vi "get_ROIs_in_um.vi"(4 "error in (no error)":errorcluster, 6 "Container State":T10, 7 "Display State In":T1={"current frame index"=0, "number of images"=0, "ROI (frames)"={"ROI"=[]}, "control refs"={"frame"=refnum, "image"=refnum, "saveROIsButton"=refnum, "loadImageSwitch"=refnum, "loadROIsSwitch"=refnum, "saveROIsSwitch"=refnum, "loadImagePath"=refnum, "loadROIPath"=refnum, "redraw"=refnum}, "calibration"={"x"=0.0, "y"=0.0, "x unit"=enum."um", "y unit"=enum."um"}, "xpaths"={"x offset"="", "y offset"="", "z offset"=""}, "offset"=refnum, "XML description"="", "number of ROIs"=0.0, "ROI Tool Buttons Visible"={"Zoom Tool"=TRUE, "Selection Tool"=TRUE, "Pan Tool"=TRUE, "Point Tool"=TRUE, "Line Tool"=TRUE, "Rectangle Tool"=TRUE, "Rotated Rectangle Tool"=TRUE, "Polyline Tool"=TRUE, "Polygon Tool"=TRUE, "Freehand Tool"=TRUE, "Closed Freehand Tool"=TRUE, "Ellipse Tool"=TRUE, "Annulus Tool"=TRUE}, "ROI color"=6618880, "number color"=6618880, "enable ROI numbering?"=FALSE, "selected path to save ROIs"=path "", "starting path"=path "", "array of overlays"=[], "pointCollection"=refnum, "ROImode"=enum."IMAQROIs", "selected point ID"=0.0, "point radius"=5, "point colours"=[], "PlotAreaSize"={"Width"=0, "Height"=0}, "last action"=enum."not specified"} {"array of overlays"."overlay size" min=1}) -> (0 "error out":errorcluster, 2 "Value":T11, 3 "Display State Out":T1={"current frame index"=0, "number of images"=0, "ROI (frames)"={"ROI"=[]}, "control refs"={"frame"=refnum, "image"=refnum, "saveROIsButton"=refnum, "loadImageSwitch"=refnum, "loadROIsSwitch"=refnum, "saveROIsSwitch"=refnum, "loadImagePath"=refnum, "loadROIPath"=refnum, "redraw"=refnum}, "calibration"={"x"=0.0, "y"=0.0, "x unit"=enum."um", "y unit"=enum."um"}, "xpaths"={"x offset"="", "y offset"="", "z offset"=""}, "offset"=refnum, "XML description"="", "number of ROIs"=0.0, "ROI Tool Buttons Visible"={"Zoom Tool"=TRUE, "Selection Tool"=TRUE, "Pan Tool"=TRUE, "Point Tool"=TRUE, "Line Tool"=TRUE, "Rectangle Tool"=TRUE, "Rotated Rectangle Tool"=TRUE, "Polyline Tool"=TRUE, "Polygon Tool"=TRUE, "Freehand Tool"=TRUE, "Closed Freehand Tool"=TRUE, "Ellipse Tool"=TRUE, "Annulus Tool"=TRUE}, "ROI color"=6618880, "number color"=6618880, "enable ROI numbering?"=FALSE, "selected path to save ROIs"=path "", "starting path"=path "", "array of overlays"=[], "pointCollection"=refnum, "ROImode"=enum."IMAQROIs", "selected point ID"=0.0, "point radius"=5, "point colours"=[], "PlotAreaSize"={"Width"=0, "Height"=0}, "last action"=enum."not specified"} {"array of overlays"."overlay size" min=1})   [LabVIEW 2010, in "XImage.xctl"]
uses:
  XImage.xctl
  <vilib>/_xctls/Container State.ctl
  ROImicrons_frames_cluster.ctl
  ROImicrons_cluster.ctl
  state.ctl
  classes/SpaceVector/SpaceVector/SpaceVector.lvclass
  classes/PointCollection/PointCollection/PointCollection.lvclass
  ROI_frames_cluster.ctl
  control_refs_cluster.ctl
  calibration_cluster.ctl
  enumerations/unit.ctl
  xpath_cluster.ctl
  overlays_cluster.ctl
  ROI_mode_enum.ctl
  last_action_enum.ctl
  <vilib>/_xctls/XControlSupport.lvlib
  classes/Image/Image/Image.lvclass
panel:
  # "Replace the Value Indicator below with an Indicator of desired type.\nDo not remove this Indicator or the others from the connector pane. \nDo not change the connector pane pattern.\nThe Value Indicator should always be the second terminal from top on the output side in the connector pane."
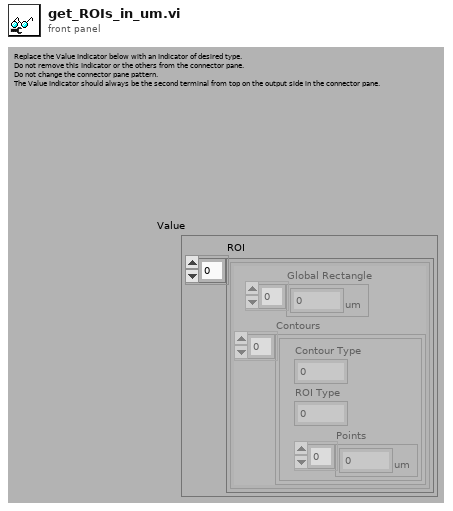
[diagram p1: front panel]
types:
  T1 = typedef "XImage.xctl/state.ctl" = cluster{"current frame index":i32, "number of images":i32, "ROI (frames)":T2, "control refs":T3, "calibration":T4, "xpaths":T6, "offset":refnum<class "SpaceVector.lvclass">, "XML description":string, "number of ROIs":dbl, "ROI Tool Buttons Visible":cluster{"Zoom Tool":bool, "Selection Tool":bool, "Pan Tool":bool, "Point Tool":bool, "Line Tool":bool, "Rectangle Tool":bool, "Rotated Rectangle Tool":bool, "Polyline Tool":bool, "Polygon Tool":bool, "Freehand Tool":bool, "Closed Freehand Tool":bool, "Ellipse Tool":bool, "Annulus Tool":bool}, "ROI color":u32, "number color":u32, "enable ROI numbering?":bool, "selected path to save ROIs":path, "starting path":path, "array of overlays":T7[], "pointCollection":refnum<class "PointCollection.lvclass">, "ROImode":T8, "selected point ID":dbl, "point radius":i32, "point colours":u32[], "PlotAreaSize":cluster{"Width":u32, "Height":u32}, "last action":T9}
  T2 = typedef "XImage.xctl/ROI_frames_cluster.ctl" = cluster{"ROI":cluster{"Global Rectangle":i32[], "Contours":cluster{"Contour Type":u32, "ROI Type":u32, "Points":i32[]}[]}[]}
  T3 = typedef "XImage.xctl/control_refs_cluster.ctl" = cluster{"frame":refnum<vi>, "image":refnum<vi>, "saveROIsButton":refnum<vi>, "loadImageSwitch":refnum<vi>, "loadROIsSwitch":refnum<vi>, "saveROIsSwitch":refnum<vi>, "loadImagePath":refnum<vi>, "loadROIPath":refnum<vi>, "redraw":refnum<vi>}
  T4 = typedef "XImage.xctl/calibration_cluster.ctl" = cluster{"x":dbl, "y":dbl, "x unit":T5, "y unit":T5}
  T5 = typedef "Image.lvclass/unit.ctl" = enum16{"um", "s"}
  T6 = typedef "XImage.xctl/xpath_cluster.ctl" = cluster{"x offset":string, "y offset":string, "z offset":string}
  T7 = typedef "XImage.xctl/overlays_cluster.ctl" = cluster{"overlay array":cluster{i32[][]}[], "overlay name":string, "color (red)":u32, "overlay size":i32, "overlay type":enum16{"crosshair", "circle"}}
  T8 = typedef "XImage.xctl/ROI_mode_enum.ctl" = enum16{"none", "IMAQROIs", "PointCollection"}
  T9 = typedef "XImage.xctl/last_action_enum.ctl" = enum16{"not specified", "image loaded", "frame changed", "ROIs changed"}
  T10 = typedef "XControlSupport.lvlib/Container State.ctl" = cluster{"Indicator?":bool, "Run Mode?":bool, " Refnum":refnum<vi>}
  T11 = typedef "XImage.xctl/ROImicrons_frames_cluster.ctl" = cluster{"ROI":T12[]}
  T12 = typedef "ROImicrons_cluster.ctl" = cluster{"Global Rectangle":dbl[unit][], "Contours":cluster{"Contour Type":u32, "ROI Type":u32, "Points":dbl[unit][]}[]}
  T13 = cluster{"Global Rectangle":dbl[unit][], "Contours":cluster{"Contour Type":u32, "ROI Type":u32, "Points":dbl[unit][]}[]}
  T14 = cluster{"Contour Type":u32, "ROI Type":u32, "Points":dbl[unit][]}
  T15 = cluster{"Global Rectangle":i32[], "Contours":cluster{"Contour Type":u32, "ROI Type":u32, "Points":i32[]}[]}[]
  T16 = cluster{"Global Rectangle":dbl[unit][], "Contours":cluster{"Contour Type":u32, "ROI Type":u32, "Points":dbl[unit][]}[]}[]
  T17 = cluster{"Contour Type":u32, "ROI Type":u32, "Points":i32[]}[]
  T18 = cluster{"[0]":dbl, "[1]":dbl, "[2]":dbl, "[3]":dbl}
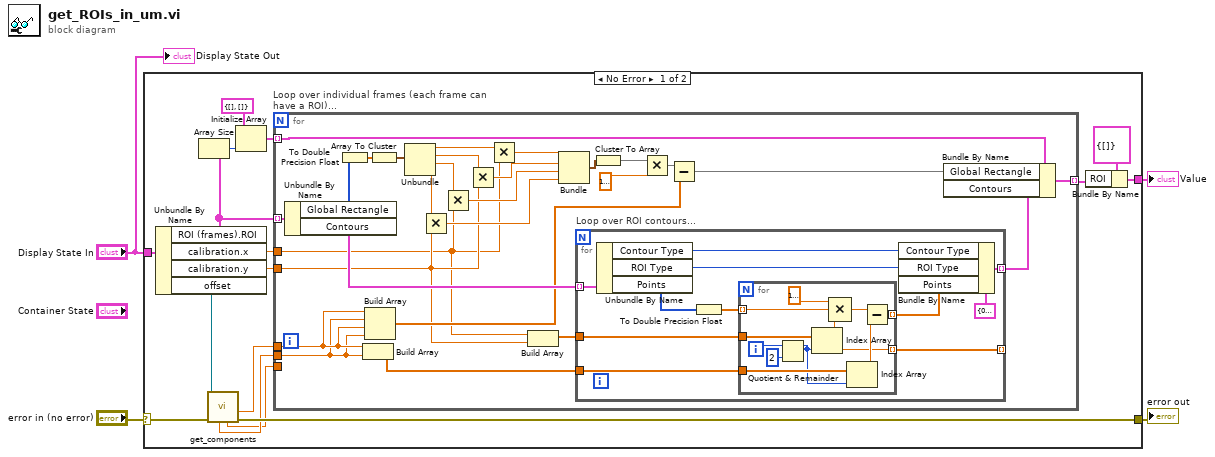
[diagram p0: block diagram]
diagram:
  n1 = case shown="No Error" "error in (no error)" {
    selector: "error in (no error)" -> [w10 w71]
    tunnel: "Display State In" -> [w20 _]
    tunnel: [w11 _] -> w3
    tunnel: [w9 w71] -> w1
    frame No Error {
      n2 = Unbundle By Name(w20) -> ("ROI (frames).ROI"=w16:T15, "calibration.x"=w19:dbl, "calibration.y"=w18:dbl, "offset"=w8:refnum<class "SpaceVector.lvclass">)
      n3 = Array Size(array=w16) -> (size(s)=w15:i32)
      n4 = call "get_components.vi"("error in (no error)"=w10, "SpaceVector in"=w8) -> ("error out"=w9:errorcluster, "x"=w7:dbl[unit], "z"=w5:dbl[unit], "y"=w6:dbl[unit])  [unwired: 4 in, 2 out]
      n5 = Initialize Array(T13 {"Global Rectangle"=[], "Contours"=[]} ("ROI"), w15) -> (w14:T16)
      n6 = for "Loop over individual frames (each frame can have a ROI)..." {
        tunnel: w16 -> [w48] mode=indexing
        tunnel: w19 -> [w21]
        tunnel: w18 -> [w22]
        tunnel: w14 -> [w36] mode=indexing
        tunnel: [w33] -> w12 mode=indexing
        tunnel: w7 -> [w28]
        tunnel: w6 -> [w27]
        tunnel: w5 -> [_]
        n7 = Unbundle By Name(w48) -> ("Global Rectangle"=w47:i32[], "Contours"=w32:T17)
        n8 = To Double Precision Float(number=w47) -> (double precision float=w46:dbl[])
        n9 = Build Array(w28, w27) -> (w29:dbl[unit][])
        n10 = Build Array(w28, w27, w28, w27) -> (w24:dbl[unit][])
        n11 = Array To Cluster(array=w46) -> (cluster=w45:T18)
        n12 = Unbundle(w45) -> ("[0]"=w44:dbl, "[1]"=w43:dbl, "[2]"=w42:dbl, "[3]"=w41:dbl)
        n13 = Multiply(x=w41, y=w22) -> (x*y=w38:dbl)
        n14 = Multiply(x=w42, y=w21) -> (x*y=w39:dbl)
        n15 = Multiply(x=w43, y=w22) -> (x*y=w40:dbl)
        n16 = Multiply(x=w44, y=w21) -> (x*y=w30:dbl)
        n17 = Build Array(w21, w22) -> (w23:dbl[])
        n18 = Bundle(w30, w40, w39, w38) -> (w37:cluster{dbl, dbl, dbl, dbl})  [unwired: 1 in]
        n19 = for "Loop over ROI contours..." {
          tunnel: w32 -> [w59] mode=indexing
          tunnel: [w54] -> w31 mode=indexing
          tunnel: w29 -> [w51]
          tunnel: w23 -> [w52]
          tunnel: [w49] -> _ mode=indexing
          n20 = Unbundle By Name(w59) -> ("Contour Type"=w56:u32, "ROI Type"=w55:u32, "Points"=w58:i32[])
          n21 = To Double Precision Float(number=w58) -> (double precision float=w53:dbl[])
          n22 = for {
            tunnel: w53 -> [w70] mode=indexing
            tunnel: w52 -> [w66]
            tunnel: w51 -> [w65]
            tunnel: [w61] -> w50 mode=indexing
            tunnel: [w60] -> w49 mode=indexing
            i -> [w68]
            n23 = Quotient & Remainder(x=w68, y=2) -> (x-y*floor(x/y)=w64:i32)  [unwired: 1 out]
            n24 = Index Array(array=w66, index=w64) -> (element=w60:dbl)
            n25 = Compound Arithmetic op=MULTIPLY(dbl[unit] 1e-06 ("x*y"), w70, w60) -> (w69:dbl[unit])
            n26 = Index Array(array=w65, index=w64) -> (element=w62:dbl[unit])
            n27 = Subtract(x=w69, y=w62) -> (x-y=w61:dbl[unit])
          }
          n28 = Bundle By Name(cluster=T14 {"Contour Type"=0, "ROI Type"=0, "Points"=[]}, "Contour Type"=w56, "ROI Type"=w55, "Points"=w50) -> (w54:T14)
        }
        n29 = Cluster To Array(cluster=w37) -> (array=w35:dbl[])
        n30 = Multiply(x=w35, y=dbl[unit] 1e-06 ("x*y")) -> (x*y=w26:dbl[unit][])
        n31 = Subtract(x=w26, y=w24) -> (x-y=w25:dbl[unit][])
        n32 = Bundle By Name(cluster=w36, "Global Rectangle"=w25, "Contours"=w31) -> (w33:T13)
      }
      n33 = Bundle By Name(cluster=T11 {"ROI"=[]} ("ROI (frames)"), "ROI"=w12) -> (w11:T11)
    }
    frame Error {
    }
  }
  "error out" <- w1
  "Value" <- w3
  "Display State Out" <- "Display State In"
